vi "DT_Triangle Manager_Get Adj_by Point.vi"(9 "point idx":i32, 10 "triangle":i32, 11 "Triangles In":i32[][](array[numeric])) -> (2 "adj triangle":i32)   [LabVIEW 2020, in "NI_AAL_Geometry.lvlib"]
uses:
  <vilib>/Analysis/NI_AAL_Geometry.lvlib
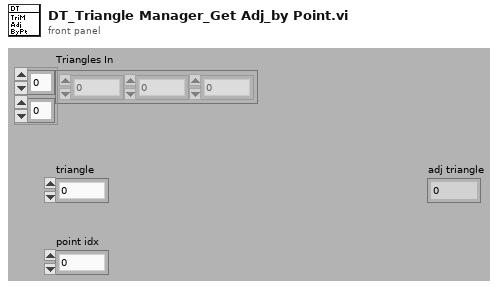
[diagram p1: front panel]
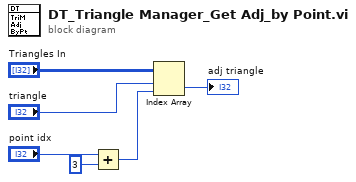
[diagram p0: block diagram]
diagram:
  n1 = Add(x="point idx", y=3) -> (x+y=w3:i32)
  n2 = Index Array(array="Triangles In", index (row)="triangle", index (col)=w3) -> (element=→"adj triangle":i32)
